vi "GLBL AO 9265.vi"(10 "9265 AO in":T1, 11 "write_read":bool) -> (2 "9265 AO out":T1)   [LabVIEW 2020]
uses:
  controls/AO_0_3.ctl
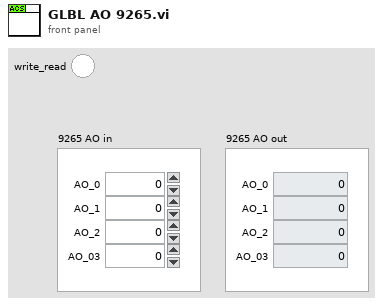
[diagram p1: front panel]
types:
  T1 = typedef "AO_0_3.ctl" = cluster{"AO_0":dbl, "AO_1":dbl, "AO_2":dbl, "AO_03":dbl}
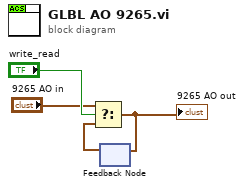
[diagram p0: block diagram]
diagram:
  n1 = feedback #1() -> (w2:T1)  [unwired: 1 in]
  n2 = Select(t="9265 AO in", s="write_read", f=w2) -> (s? t:f=w3:T1)
  "9265 AO out" <- w3
  n3 = feedback-in #1(w3) -> ()
